vi "Close.vi"(8 "error in (no error)":errorcluster, 11 "CameraLan in":refnum<class "CameraLan.lvclass">) -> (0 "error out":errorcluster)   [LabVIEW 2011, in "CameraLan.lvclass"]
uses:
  CameraLan.lvclass
  CameraLan.lvclass/CameraLan.ctl
  <vilib>/vision/driver/NI_Vision_Acquisition_Software.lvlib
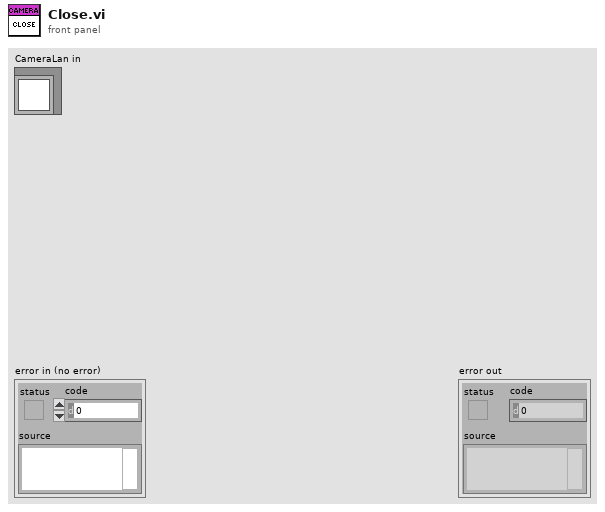
[diagram p1: front panel]
types:
  T1 = typedef "IMAQdx.ctl" = refnum<k21>
  T2 = typedef "IMAQ Image.ctl" = refnum<image>
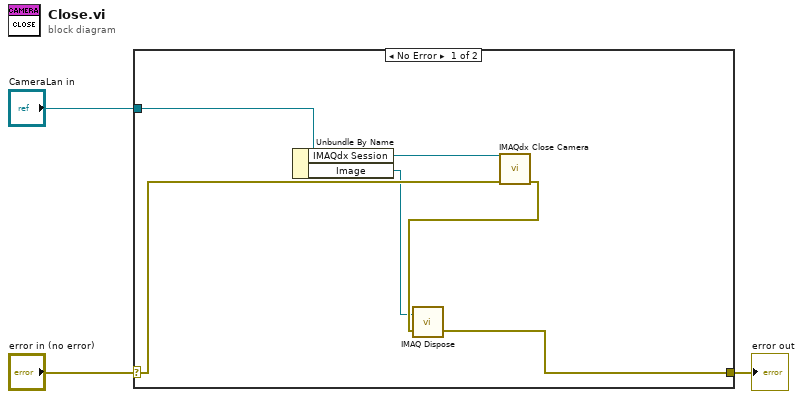
[diagram p0: block diagram]
diagram:
  n1 = case shown="No Error" "error in (no error)" {
    selector: "error in (no error)" -> [w8 w10]
    tunnel: [w5 w10] -> w2
    tunnel: "CameraLan in" -> [w9 _]
    frame No Error {
      n2 = Unbundle By Name(w9) -> ("IMAQdx Session"=w7:T1, "Image"=w4:T2)
      n3 = call <vilib>:"IMAQdx Close Camera.vi"("error in"=w8, "Session In"=w7) -> ("error out"=w6:errorcluster)  [unwired: 9 out]
      n4 = call "IMAQ Dispose"("Image"=w4, "error in (no error)"=w6) -> ("error out"=w5:errorcluster)  [unwired: 4 in]
    }
    frame Error {
    }
  }
  "error out" <- w2
